vi "GetCaseStructureByName.vi"(8 "error in (no error)":errorcluster, 10 "CaseStructureLabel.Text":string="ScriptedCaseStructure", 11 "VI Refnum":refnum<vi>) -> (0 "error out":errorcluster, 2 "CaseStructure Ref":refnum<vi>, 3 "VI Refnum":refnum<vi>)   [LabVIEW 2019, in "BlueUtilityScripts.lvlib"]
uses:
  BlueUtilityScripts.lvlib
  <vilib>/Utility/traverseref.llb/TRef TravTarget.ctl
  <userlib>/_OpenG.lib/array/array.llb/Search 1D Array (String)__ogtk.vi
  <vilib>/Utility/error.llb/Error Cluster From Error Code.vi
  <vilib>/ErrorRing/Error Ring.xnode
  <vilib>/Utility/traverseref.llb/VI Scripting - Traverse.lvlib
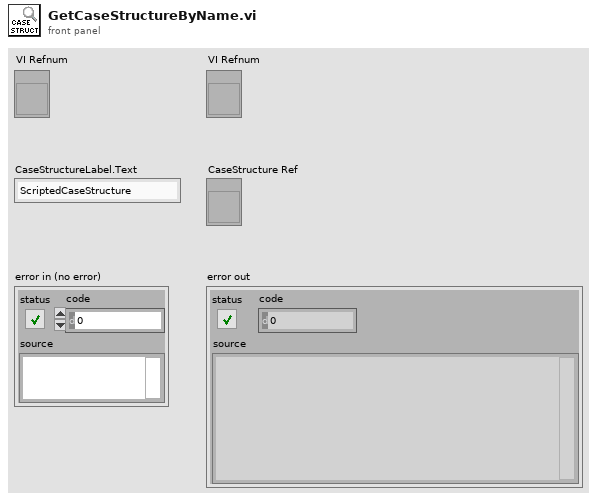
[diagram p1: front panel]
types:
  T1 = typedef "TRef TravTarget.ctl" = enum16{"FP", "BD", "Other"}
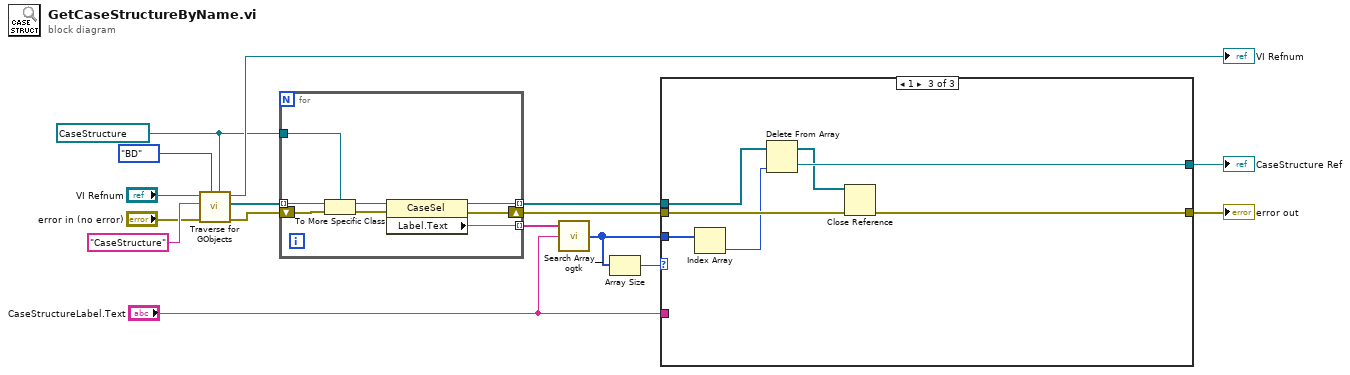
[diagram p0: block diagram]
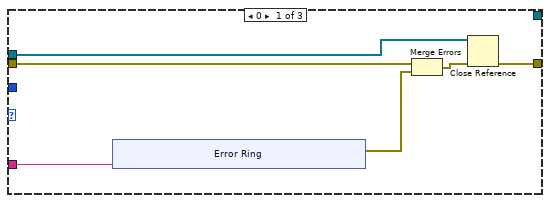
[diagram p2: hidden frame]
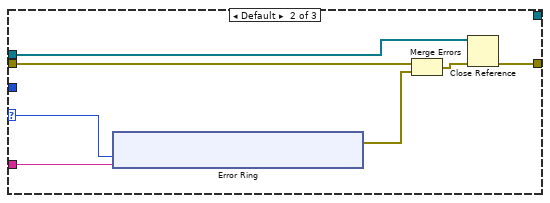
[diagram p3: hidden frame]
diagram:
  w9 = refnum<vi> refnum ("Other Refnum")
  n1 = call <vilib>:"Traverse for GObjects.vi"("Other Refnum"=w9, "Traverse Target"=TRef_TravTarget."BD", "error in (no error)"="error in (no error)", "Class Name"="CaseStructure", "VI Refnum"="VI Refnum") -> ("error out"=w8:errorcluster, "References"=w10:refnum<vi>[], "dup VI Refnum"=→"VI Refnum":refnum<vi>)  [unwired: 3 in, 1 out]
  n2 = for {
    tunnel: w10 -> [w22] mode=indexing
    tunnel: w9 -> [w21]
    shift-right: [w19] -> w7
    shift-left: w8 -> [w20]
    tunnel: [w18] -> w6 mode=indexing
    tunnel: [w17] -> w4 mode=indexing
    n3 = To More Specific Class(target class=w21, reference=w22, error in=w20) -> (specific class reference=w23:refnum<vi>, error out=w24:errorcluster)
    n4 = property class="CaseSel"(reference=w23, error in=w24) -> (reference out=w18:refnum<vi>, error out=w19:errorcluster, "Label.Text"=w17:string)
  }
  n5 = call-poly <userlib>:"Search Array__ogtk.vi"("Array"=w4, "Element Data"="CaseStructureLabel.Text") -> ("Indices of Elements"=w1:i32[])  [unwired: 7 in]
  n6 = Array Size(array=w1) -> (size(s)=w2:i32)
  n7 = case shown="1" w2 {
    selector: w2 -> [_ w38 _]
    tunnel: [w25 w40 w55] -> w11
    tunnel: w7 -> [w28 w43 w56]
    tunnel: w6 -> [w26 w41 w59]
    tunnel: "CaseStructureLabel.Text" -> [w30 w39 _]
    tunnel: [_ _ w58] -> w5
    tunnel: w1 -> [_ _ w54]
    frame 0 {
      n8 = xnode "Error Ring"("parameter 0"=w30) -> ("error out"=w29:errorcluster)
      n9 = Merge Errors(w28, w29) -> (w27:errorcluster)
      n10 = Close Reference(reference=w26, error in (no error)=w27) -> (error out=w25:errorcluster)
    }
    frame Default {
      n11 = xnode "Error Ring"("parameter 0"=w38, "parameter 1"=w39) -> ("error out"=w44:errorcluster)
      n12 = Merge Errors(w43, w44) -> (w42:errorcluster)
      n13 = Close Reference(reference=w41, error in (no error)=w42) -> (error out=w40:errorcluster)
    }
    frame 1 {
      n14 = Index Array(array=w54) -> (element=w53:i32)  [unwired: 1 in]
      n15 = Delete From Array(array=w59, index=w53) -> (deleted portion=w58:refnum<vi>, array with subset deleted=w57:refnum<vi>[])  [unwired: 1 in]
      n16 = Close Reference(reference=w57, error in (no error)=w56) -> (error out=w55:errorcluster)
    }
  }
  "error out" <- w11
  "CaseStructure Ref" <- w5
